vi "2100_Bridge_Read RFFE_w_Waveform.vi"(0 "Semiconductor Module Context":T2, 1 "USID":T1 max=15, 2 "Reg Address":u8=31, 5 "Pins":string[](array[string])=["CLK", "SDA"], 7 "Reg_Map":string[][](array[string])=[["Reg Addr(0x00)", "7", "6", "5", "4", "3", "2", "1", "0"], ["0", "SPARE", "RF3_SH", "RF2_SH", "RF1_SH", "SPARE", "RF3_RFC", "RF2_RFC", "RF1_RFC"], ["1", "SPARE[7:0]", "", "", "", "", "", "", ""], ["2", "VVAR_EN", "LCM_EN", "RFC_SH", "SPARE", "VARACTOR[3:0]", "", "", ""], ["3", "SW_CTRL1_VIRTUAL[7:0]", "", "", "", "", "", "", ""], ["4", "SW_CTRL1_SWAP", "SW_CTRL1_RBSHIFT[2:0]", "", "", "SW_CTRL1_VSID[3:0]", "", "", ""], ["5", "REG_00_VIRTUAL_MASK[7:0]", "", "", "", "", "", "", ""], ["6", "LOCK_STATUS[1:0]", "", "CLK_DITHER", "FUSES_BURNED", "CLK_IDAC_CAL[3:0]", "", "", ""], ["7", "SPARE[2:0]", "", "", "ODFT_TRIM[4:0]", "", "", "", ""], ["8", "SPARE[2:0]", "", "", "HV_TRIM[4:0]", "", "", "", ""], ["9", "TEST_MUX[2:0]", "", "", "SPARE[1:0]", "", "MEMS_BG_TC[1:0]", "", "MEMSCP_RCM"], ["A", "CP_BOOST_OVRD_EN", "SPARE[2:0]", "", "", "PS_OFF_TIMER[1:0]", "", "PS_ON_TIMER[1:0]", ""], ["0", "", "", "", "", "", "", "", ""], ["D", "Reserved[1:0]", "", "WD_HI_EVENT_CNT[5:0]", "", "", "", "", ""], ["E", "VERSION_ID[7:0]", "", "", "", "", "", "", ""], ["F", "Reserved", "COUNT_200_LSB[6:0]", "", "", "", "", "", ""], ["10", "CLK_DIV2_EN", "Spare", "ODFT_EN", "HV_HYST[4:0]", "", "", "", ""], ["0", "", "", "", "", "", "", "", ""], ["12", "SHORT_FUSE", "FUSE_BURN", "STROBE_EN", "VIO_OK", "RTH[1:0]", "", "FUSE_LOAD_MAN_EN", "FUSE_LOAD"], ["13", "RR_ACK_EN", "Reserved", "ACK_POSITION[1:0]", "", "SuBUS_DRIVE_STRENGTH[3:0]", "", "", ""], ["14", "TM_IO_EN", "TM_IO_SEL", "SuBUS_OVS[1:0]", "", "Reserved[3:0]", "", "", ""], ["15", "Reserved[4:0]", "", "", "", "", "SuBUS_VERSION_PRESENT", "SuBUS_VOLTAGE", "SuBUS_FLAVOR_DEF"], ["16", "PROG_STROBE1_DUR[7:0]", "", "", "", "", "", "", ""], ["17", "PROG_STROBE0_DUR[7:0]", "", "", "", "", "", "", ""], ["18", "Reserved[2:0]", "", "", "EFUSE_SINGLE_ADDR_SEL[4:0]", "", "", "", ""], ["19", "POLL_ADR[4:0]", "", "", "", "", "POLL_BC[2:0]", "", ""], ["1A", "SOFTWARE_RESET", "Reserved[6:0]", "", "", "", "", "", ""], ["1B", "Reserved[7:0]", "", "", "", "", "", "", ""], ["1C", "PWR_MODE_1", "PWR_MODE_0", "TRIGGER_MASK[2:0]", "", "", "TRIGGER[2:0]", "", ""], ["1D", "PRODUCT_ID[7:0]", "", "", "", "", "", "", ""], ["1E", "MANUFACTURER_ID_LSB[7:0]", "", "", "", "", "", "", ""], ["1F", "MANUFACTURER_ID_MSB[3:0]", "", "", "", "USID[3:0]", "", "", ""]], 9 "Reg_Map_Bit_Name":string="HV_TRIM", 11 "Error In":errorcluster, 13 "Publish_Data?":bool, 14 "Published Data Id":string) -> (4 "Converted Data":T3 {"Register" max=31 format="%.0x"; "Slave Address" max=15 format="%.0x"}, 6 "Bit Value":u8 format="%.0b", 15 "Error Out":errorcluster)   [LabVIEW 2013]
uses:
  <vilib>/NI_TestStand_SemiconductorModule/NI_TestStand_Semiconductor_Module.lvlibp/PinMap/General/SemiconductorModuleContext.ctl
  Controls/USID.ctl
  Controls/Reg_Address_Data.ctl
  <vilib>/NI_TestStand_SemiconductorModule/NI_TestStand_Semiconductor_Module.lvlibp
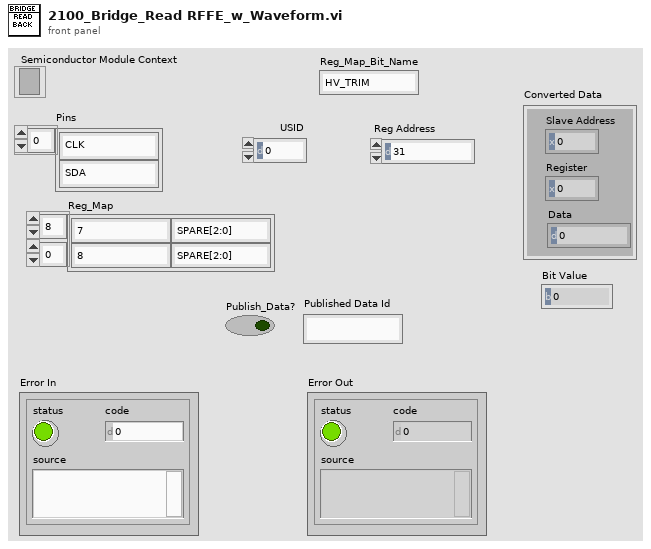
[diagram p1: front panel]
types:
  T1 = typedef "USID.ctl" = u8
  T2 = typedef "NI_TestStand_Semiconductor_Module.lvlibp/SemiconductorModuleContext.ctl" = refnum<k7>
  T3 = cluster{"Slave Address":u8, "Register":u8, "Data":u8}
  T4 = typedef "Reg_Address_Data.ctl" = cluster{"Address":u8, "Data":u8}
  T5 = cluster{"First Reg Address":u8, "Num of Reg to Read":u8}
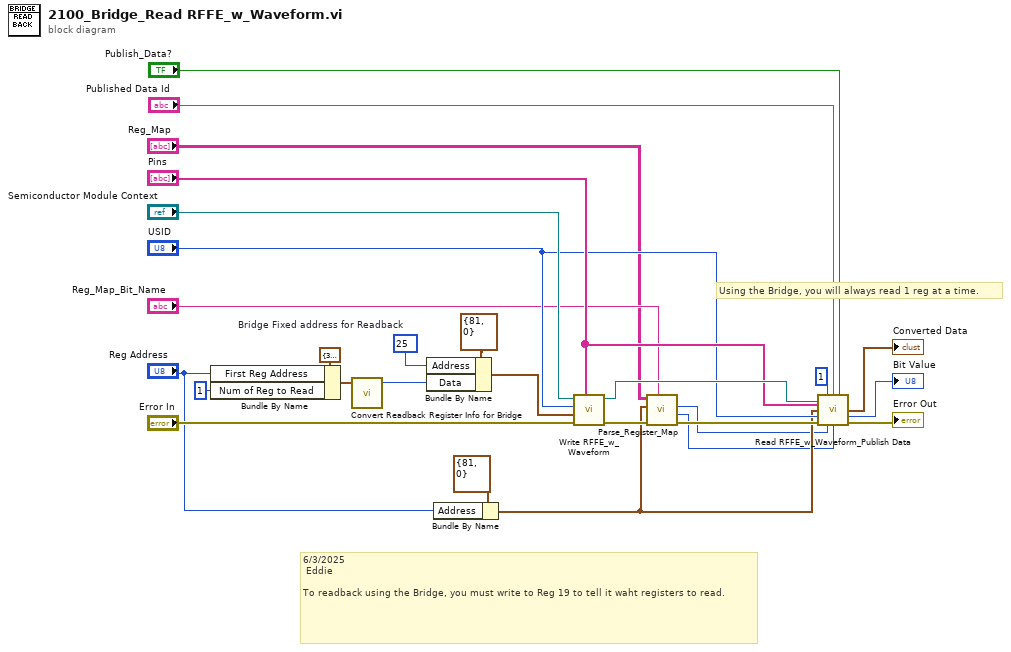
[diagram p0: block diagram]
diagram:
  w25 = u8 25  # Bridge Fixed address for Readback
  # "Using the Bridge, you will always read 1 reg at a time."
  # "6/3/2025\n Eddie\n\nTo readback using the Bridge, you must write to Reg 19 to tell it waht registers to read."
  n1 = Bundle By Name(cluster=T5 {"First Reg Address"=31, "Num of Reg to Read"=31} ("Reg_Address_to_Read"), "First Reg Address"="Reg Address", "Num of Reg to Read"=u8 1) -> (w14:T5)
  n2 = call "Convert Readback Register Info for Bridge.vi"("Reg_Address_to_Read"=w14) -> ("number"=w26:u32)  [unwired: 4 in]
  n3 = Bundle By Name(cluster=T4 {"Address"=81, "Data"=0} ("Reg_Address_Data"), "Address"=w25, "Data"=w26) -> (w23:T4)
  n4 = Bundle By Name(cluster=T4 {"Address"=81, "Data"=0} ("Reg_Address_Data"), "Address"="Reg Address") -> (w6:T4)
  n5 = call "Write RFFE_w_Waveform.vi"("Pins"="Pins", "error in (no error)"="Error In", "Reg_Address_Data"=w23, "USID"="USID", "Semiconductor Module Context"="Semiconductor Module Context") -> ("error out"=w10:errorcluster, "Semiconductor Module Context Out"=w21:T2)  [unwired: 5 in]
  n6 = call "Parse_Register_Map.vi"("Reg_Map_Bit_Name"="Reg_Map_Bit_Name", "Error In"=w10, "Reg_Address_Data"=w6, "Reg_Map"="Reg_Map") -> ("Error Out"=w9:errorcluster, "Length"=w4:u8, "LSB"=w5:u8)  [unwired: 4 in, 1 out]
  n7 = call "Read RFFE_w_Waveform_Publish Data.vi"("Semiconductor Module Context"=w21, "Num_Reg_to_Read"=u8 1, "Published Data Id"="Published Data Id", "Publish_Data?"="Publish_Data?", "Pins"="Pins", "Reg_Address_Data"=w6, "USID"="USID", "Error In"=w9, "Bit_Location(LSB)"=w5, "#ofBits"=w4) -> ("Converted Data"=→"Converted Data":T3, "Reg Value"=→"Bit Value":u8, "Error Out"=→"Error Out":errorcluster)  [unwired: 1 in, 2 out]
